vi "Timer Test (SubVI).vi"(8 "Error In":errorcluster, 10 "Boolean":bool) -> (0 "Error Out":errorcluster, 2 "t":dbl)   [LabVIEW 2020]
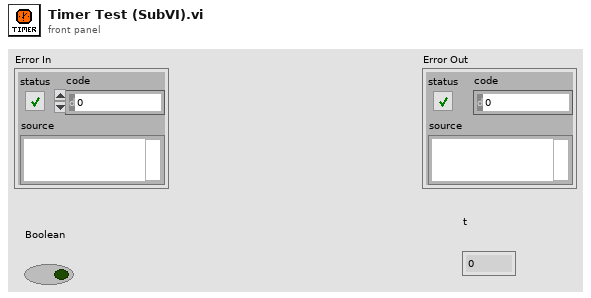
[diagram p1: front panel]
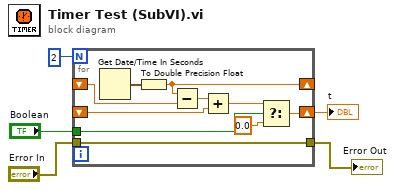
[diagram p0: block diagram]
diagram:
  n1 = for {
    N: 2 -> [_]
    shift-right: [w13] -> _
    shift-left: _ -> [w14]
    shift-right: [w11] -> w4
    shift-left: _ -> [w10]
    tunnel: "Boolean" -> [w9]
    tunnel: "Error In" -> [w6]
    tunnel: [w6] -> w1
    n2 = Get Date/Time In Seconds() -> (seconds since 1Jan1904=w15:timestamp)
    n3 = To Double Precision Float(number=w15) -> (double precision float=w13:dbl)
    n4 = Subtract(x=w13, y=w14) -> (x-y=w12:dbl)
    n5 = Add(x=w12, y=w10) -> (x+y=w7:dbl)
    n6 = Select(t=w7, s=w9, f=0.0 ("t")) -> (s? t:f=w11:dbl)
  }
  "t" <- w4
  "Error Out" <- w1
